vi "Dynamic call-Funct img TIFF exporter.vi"(8 "error in (no error)":errorcluster) -> (0 "error out":errorcluster)   [LabVIEW 2020]
uses:
  Processing/Patches/Globals/gl_funct TIFF export globals.vi
panel:
  out "appended path":path
  out "Funct TIFF export-Window is open":bool
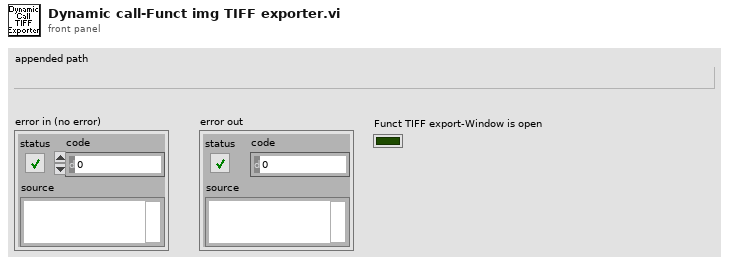
[diagram p1: front panel]
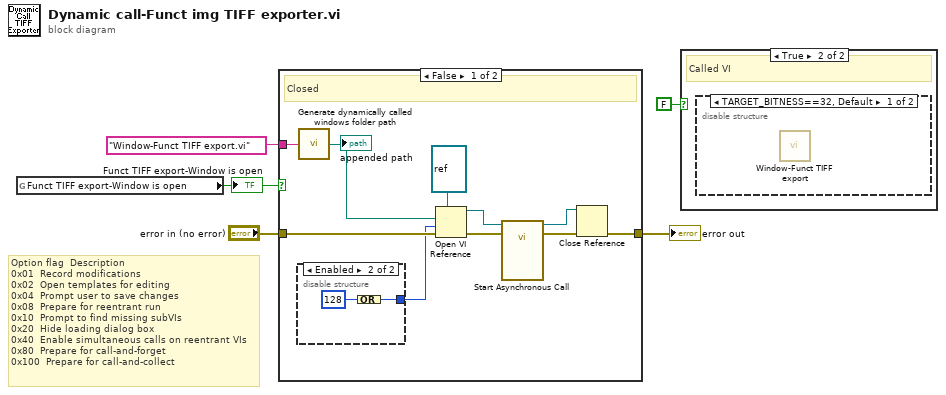
[diagram p0: block diagram]
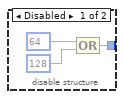
[diagram p4: hidden frame]
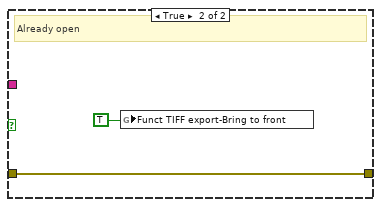
[diagram p5: hidden frame]
diagram:
  # "Option flag \tDescription\n0x01 \tRecord modifications\n0x02 \tOpen templates for editing\n0x04 \tPrompt user to save changes\n0x08 \tPrepare for reentrant run\n0x10 \tPrompt to find missing subVIs\n0x20 \tHide loading dialog box\n0x40 \tEnable simultaneous calls on reentrant VIs\n0x80 \tPrepare for call-and-forget\n0x100 \tPrepare for call-and-collect"
  n1 = global read "gl_funct TIFF export globals.vi" "Funct TIFF export-Window is open"() -> (w3:bool)
  "Funct TIFF export-Window is open" <- w3
  n2 = case shown="False" w3 {
    tunnel: "error in (no error)" -> [w15 w22]
    tunnel: [w14 w22] -> w4
    tunnel: "Window-Funct TIFF export.vi" ("Error Source") -> [w6 _]
    frame False {
      # "Closed"
      n3 = disable-structure shown="Enabled" {
        disable-tunnel: [w18 w20] -> w11
        frame Disabled {
          n4 = Compound Arithmetic op=OR(64, 128) -> (w18:i32)
        }
        frame Enabled {
          n5 = Compound Arithmetic op=OR(128) -> (w20:i32)
        }
      }
      n6 = call "Generate dynamically called windows folder path.vi"("name of dynamically called VI"=w6) -> ("Dynamically called VI path"=w7:path)
      "appended path" <- w7
      n7 = Open VI Reference(type specifier VI Refnum (for type only)=refnum<vi> refnum, vi path=w7, options=w11, error in (no error)=w15) -> (vi reference=w12:refnum<vi>, error out=w13:errorcluster)  [unwired: 2 in]
      n8 = call-by-ref "Start Asynchronous Call"(reference=w12, error in=w13) -> (reference out=w8:refnum<vi>, error out=w9:errorcluster)  [unwired: 12 in]
      n9 = Close Reference(reference=w8, error in (no error)=w9) -> (error out=w14:errorcluster)
    }
    frame True {
      # "Already open"
      n10 = global write "gl_funct TIFF export globals.vi" "Funct TIFF export-Bring to front"(TRUE ("Bring Timelapse Editor to front")) -> ()
    }
  }
  "error out" <- w4
  n11 = case shown="True" FALSE {
    frame False {
    }
    frame True {
      # "Called VI"
      n12 = disable-structure shown="TARGET_BITNESS==32, Default" {
        frame condition #0 {
          n13 = call "Window-Funct TIFF export.vi"() -> ()  [unwired: 12 in]
        }
        frame condition #1 (active) {
        }
      }
    }
  }
